vi "Explain Error_Status Flag.vi"(11 "Error/Status Flag":i16) -> (3 "Expalined Flag":T1)   [LabVIEW 2017, in "NI_Robotics_KUKA youBot Host.lvlib"]
uses:
  <vilib>/robotics/KUKA youBot/NI_Robotics_KUKA youBot Host.lvlib
  <vilib>/robotics/KUKA youBot/EtherCAT/CmdCtrls/Error_Status Flag.ctl
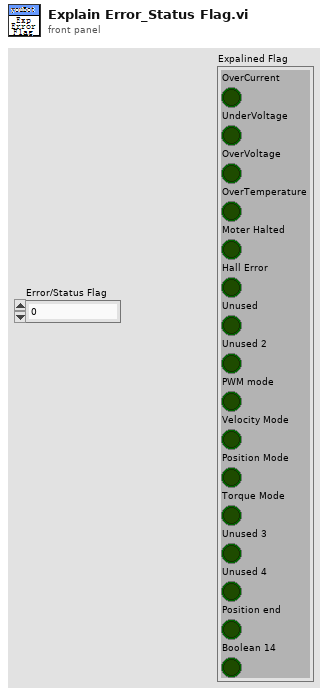
[diagram p1: front panel]
types:
  T1 = typedef "NI_Robotics_KUKA youBot Host.lvlib/Error_Status Flag.ctl" = cluster{"OverCurrent":bool, "UnderVoltage":bool, "OverVoltage":bool, "OverTemperature":bool, "Moter Halted":bool, "Hall Error":bool, "Unused":bool, "Unused 2":bool, "PWM mode":bool, "Velocity Mode":bool, "Position Mode":bool, "Torque Mode":bool, "Unused 3":bool, "Unused 4":bool, "Position end":bool, "Boolean 14":bool}
  T2 = cluster{"Boolean array[0]":bool, "Boolean array[1]":bool, "Boolean array[2]":bool, "Boolean array[3]":bool, "Boolean array[4]":bool, "Boolean array[5]":bool, "Boolean array[6]":bool, "Boolean array[7]":bool, "Boolean array[8]":bool, "Boolean array[9]":bool, "Boolean array[10]":bool, "Boolean array[11]":bool, "Boolean array[12]":bool, "Boolean array[13]":bool, "Boolean array[14]":bool, "Boolean array[15]":bool}
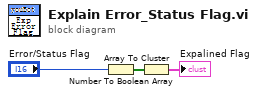
[diagram p0: block diagram]
diagram:
  n1 = Number To Boolean Array(number="Error/Status Flag") -> (Boolean array=w2:bool[])
  n2 = Array To Cluster(array=w2) -> (cluster=→"Expalined Flag":T2)
